vi "Element Init.vi"(7 "VolatusAPI":refnum<class "VolatusAPI.lvclass">, 8 "error in (no error)":errorcluster, 10 "JSON":string, 11 "GuiLinkButton in":refnum<class "GuiLinkButton.lvclass">) -> (0 "error out":errorcluster, 3 "GuiLinkButton out":refnum<class "GuiLinkButton.lvclass">)   [LabVIEW 2020, in "VolatusGUIElements.lvlib" / "GuiLinkButton.lvclass"]
uses:
  GuiLinkButton.lvclass
  GuiLinkButton.lvclass/GuiLinkButton.ctl
  1d63baae-acb0-4f4e-88fb-e1bed0605d47.vi
  JSON.ctl
  Volatus/VolatusAPI/VolatusAPI.lvclass
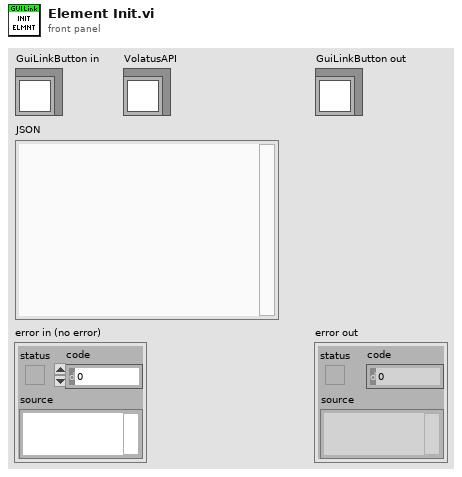
[diagram p1: front panel]
types:
  T1 = typedef "VolatusGUIElements.lvlib/GuiLinkButton.lvclass/JSON.ctl" = cluster{"ID":string}
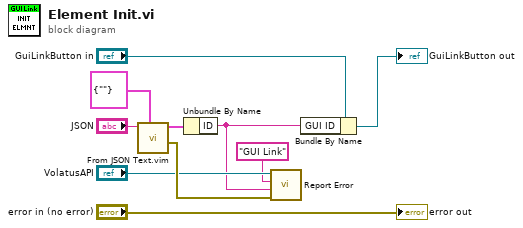
[diagram p0: block diagram]
diagram:
  n1 = call "From JSON Text.vim"("Data Type and Default Value"=T1 {"ID"=""} ("JSON"), "JSON"="JSON") -> ("error out"=w10:errorcluster, "Data out"=w5:T1)  [unwired: 8 in]
  n2 = Unbundle By Name(w5) -> ("ID"=w1:string)
  n3 = call "Report Error.vi"("error in (no error)"=w10, "Message"=w1, "Context"="GUI Link", "VolatusAPI in"="VolatusAPI") -> ()  [unwired: 6 in, 2 out]
  n4 = Bundle By Name(cluster="GuiLinkButton in", "GUI ID"=w1) -> (→"GuiLinkButton out":refnum<class "GuiLinkButton.lvclass">)
  "error out" <- "error in (no error)"
